vi "Seial Check.vi"() -> ()   [LabVIEW 2015]
uses:
  <vilib>/Instr/_visa.llb/VISA Configure Serial Port (Instr).vi
panel:
  out "String":string
  in  "stop":bool
  in  "VISA resource name":refnum<visa-resource-name>
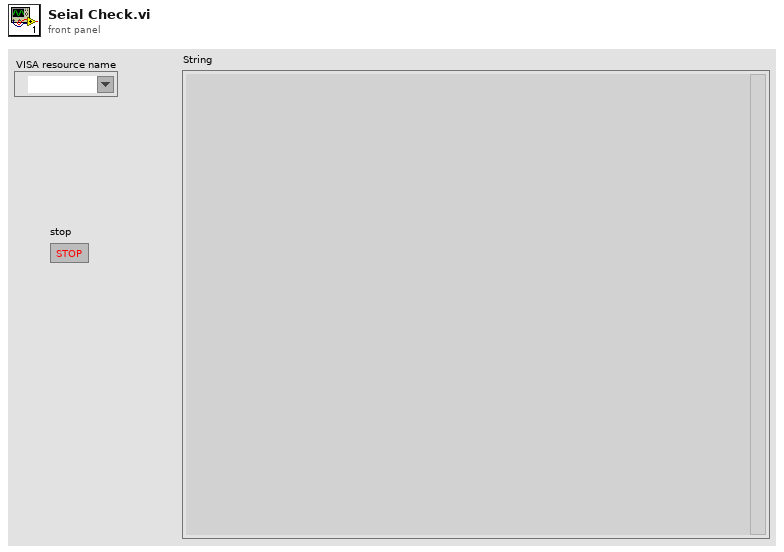
[diagram p1: front panel]
types:
  T1 = cluster{"Time Stamp":timestamp, "A":string, "B":string, "C":string}
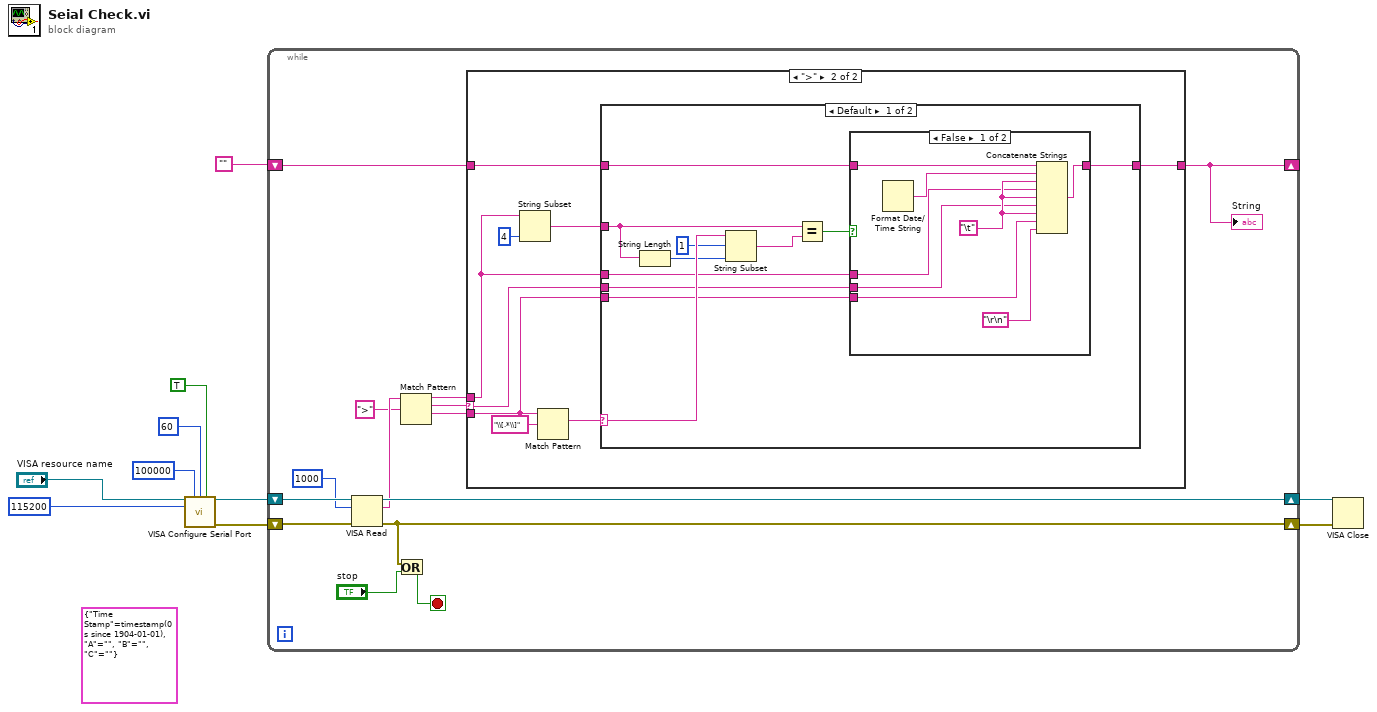
[diagram p0: block diagram]
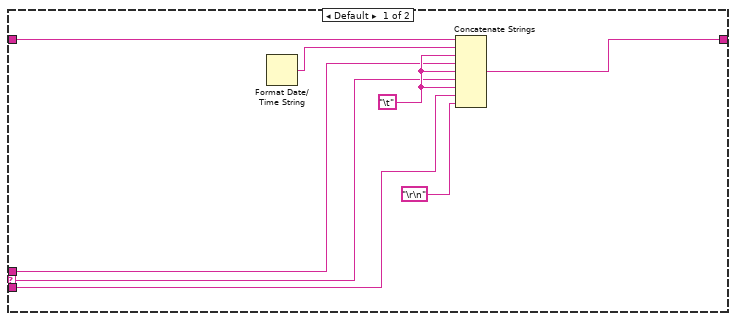
[diagram p2: hidden frame]
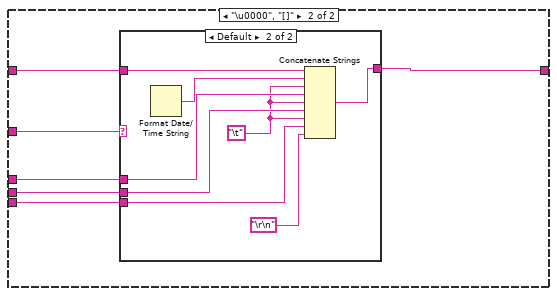
[diagram p4: hidden frame]
diagram:
  (unwired) T1 {"Time Stamp"=timestamp(0 s since 1904-01-01), "A"="", "B"="", "C"=""} ("Cluster")
  n1 = call-poly "VISA Configure Serial Port"("VISA resource name"="VISA resource name", "timeout (10sec)"=u32 100000, "termination char\n(0xA = '\\n' = LF)"=u8 60 ("termination char\n(0xA = '\\n' = LF)"), "Enable Termination\nChar (T)"=TRUE ("Enable Termination\nChar (T)"), "baud rate (9600)"=u32 115200) -> ("VISA resource name out"=w7:refnum<visa-resource-name>, "error out"=w6:errorcluster)  [unwired: 9 in]
  n2 = while {
    shift-right: [w21] -> w3
    shift-left: w7 -> [w24]
    shift-right: [w11] -> w4
    shift-left: w6 -> [w23]
    shift-right: [w14] -> _
    shift-left: "" -> [w15]
    stop <- w13 stop-if-true
    n3 = VISA Read(VISA resource name=w24, byte count=u32 1000, error in (no error)=w23) -> (VISA resource name out=w21:refnum<visa-resource-name>, read buffer=w20:string, error out=w11:errorcluster)  [unwired: 1 out]
    n4 = Or(x=w11, y="stop") -> (x .or. y?=w13:bool)
    n5 = Match Pattern(string=w20, regular expression=">") -> (before substring=w17:string, match substring=w18:string, after substring=w16:string)  [unwired: 1 in, 1 out]
    n6 = case shown="\">\"" w18 {
      selector: w18 -> [w26 w36]
      tunnel: w17 -> [w25 w34]
      tunnel: w16 -> [w27 w37]
      tunnel: w15 -> [w29 w38]
      tunnel: [w28 w39] -> w14
      frame Default {
        w31 = "\t"
        n7 = Format Date/Time String() -> (date/time string=w32:string)  [unwired: 3 in]
        n8 = Concatenate Strings(w29, w32, w31, w25, w31, w26, w31, w27, "\r\n") -> (w28:string)
      }
      frame ">" {
        n9 = String Subset(string=w34, length (rest)=4 ("length (rest)")) -> (substring=w33:string)  [unwired: 1 in]
        n10 = Match Pattern(string=w37, regular expression="\\[.*\\]") -> (match substring=w40:string)  [unwired: 1 in, 3 out]
        n11 = case shown="Default" w40 {
          selector: w40 -> [w52 _]
          tunnel: [w49 w64] -> w39
          tunnel: w38 -> [w50 w65]
          tunnel: w37 -> [w46 w66]
          tunnel: w36 -> [w47 w67]
          tunnel: w34 -> [w48 w63]
          tunnel: w33 -> [w43 w62]
          frame Default {
            n12 = String Length(string=w43) -> (length=w42:i32)
            n13 = String Subset(string=w52, offset (0)=1, length (rest)=w42) -> (substring=w51:string)
            n14 = Equal?(x=w43, y=w51) -> (x = y?=w45:bool)
            n15 = case shown="False" w45 {
              tunnel: w50 -> [w57 w61]
              tunnel: [w56 w61] -> w49
              tunnel: w48 -> [w55 _]
              tunnel: w47 -> [w54 _]
              tunnel: w46 -> [w53 _]
              frame False {
                w59 = "\t"
                n16 = Format Date/Time String() -> (date/time string=w60:string)  [unwired: 3 in]
                n17 = Concatenate Strings(w57, w60, w59, w55, w59, w54, w59, w53, "\r\n") -> (w56:string)
              }
              frame True {
              }
            }
          }
          frame "\u0000", "[]" {
            n18 = case shown="Default" w62 {
              tunnel: w67 -> [_ w72]
              tunnel: w66 -> [_ w71]
              tunnel: w65 -> [w68 w76]
              tunnel: [w68 w75] -> w64
              tunnel: w63 -> [_ w73]
              frame "led2" {
              }
              frame Default {
                w70 = "\t"
                n19 = Format Date/Time String() -> (date/time string=w74:string)  [unwired: 3 in]
                n20 = Concatenate Strings(w76, w74, w70, w73, w70, w72, w70, w71, "\r\n") -> (w75:string)
              }
            }
          }
        }
      }
    }
    "String" <- w14
  }
  n21 = VISA Close(VISA resource name=w3, error in (no error)=w4) -> ()  [unwired: 1 out]
